vi "Convert-speed.vi"(8 "error in (no error)":errorcluster, 10 "Speed in":dbl caption="Speed [unit/s]", 11 "Motor-Serial in":refnum<class "Motor-Serial.lvclass">) -> (0 "error out":errorcluster, 2 "Speed out":dbl caption="Speed out [rpm]", 3 "Motor-Serial out":refnum<class "Motor-Serial.lvclass">)   [LabVIEW 2013, in "PowderDeposition.lvlib" / "Motor-Serial.lvclass"]
uses:
  Motor-Serial.lvclass
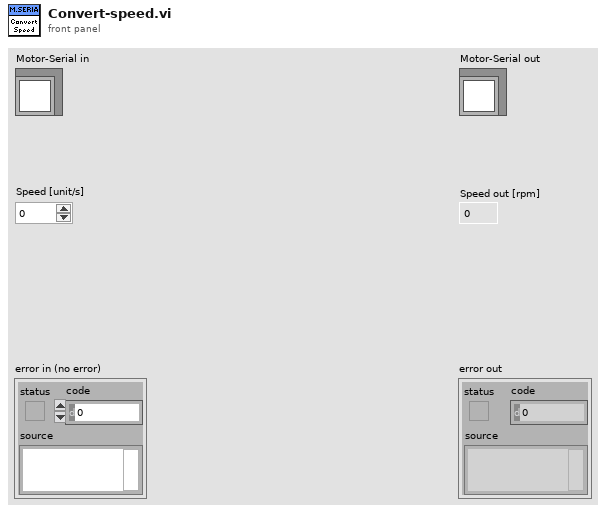
[diagram p1: front panel]
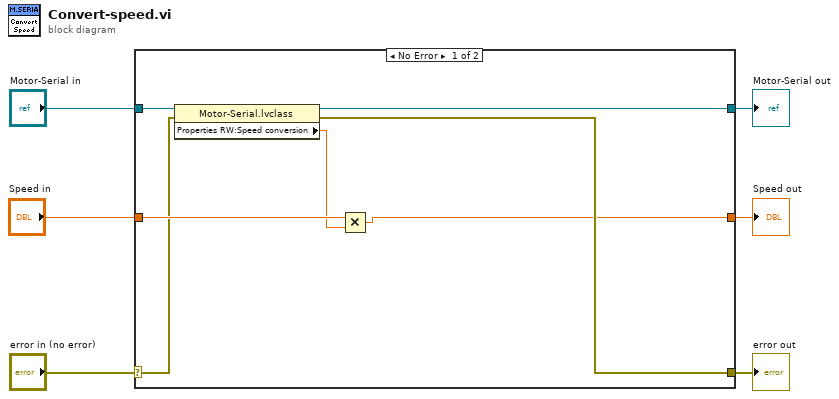
[diagram p0: block diagram]
diagram:
  n1 = case shown="No Error" "error in (no error)" {
    selector: "error in (no error)" -> [w9 w16]
    tunnel: [w8 w16] -> w5
    tunnel: [w13 w15] -> w3
    tunnel: "Motor-Serial in" -> [w12 w15]
    tunnel: "Speed in" -> [w11 w14]
    tunnel: [w7 w14] -> w1
    frame No Error {
      n2 = property class="Motor-Serial.lvclass"(reference=w12, error in=w9) -> (reference out=w13:refnum<class "Motor-Serial.lvclass">, error out=w8:errorcluster, "Properties RW:Speed conversion"=w10:dbl)
      n3 = Multiply(x=w11, y=w10) -> (x*y=w7:dbl)
    }
    frame Error {
    }
  }
  "error out" <- w5
  "Motor-Serial out" <- w3
  "Speed out" <- w1
